vi "Vision Aim 359.vi"(11 "abort":bool) -> (0 "ARM GOOD":bool=TRUE, 1 "WHEELS GOOD":bool, 2 "Vision In Range?":bool=TRUE, 3 "Gyro":dbl=-9.742404543514061 format="%.2f")   [LabVIEW 2015]
uses:
  <vilib>/addons/control/pid/pid.llb/PID Control Input Filter (DBL).vi
  Code/Robot Global Data.vi
  <vilib>/Rock Robotics/WPI/Utilities/WPI_GetSetVariantRefNum.vi
  <vilib>/Rock Robotics/WPI/RobotDrive/WPI_RobotDriveArcadeDrive_Standard(NoSaturation).vi
  <vilib>/addons/control/pid/NI_PID_pid.lvlib
panel:
  out "Enum":T1(ring)
  out "Vision":dbl=-0.01718749999999998 format="%.2f"
  in  "Range 2":dbl=0.03
  in  "Speed 2":dbl=0.4
  in  "Speed 1":dbl=0.55
  in  "Range 1":dbl=0.2
  in  "Vision Tolerance":dbl=0.03
  # "Outputs"
  # "Turning Gains"
  # ".55\n.75\n.45\n.05"
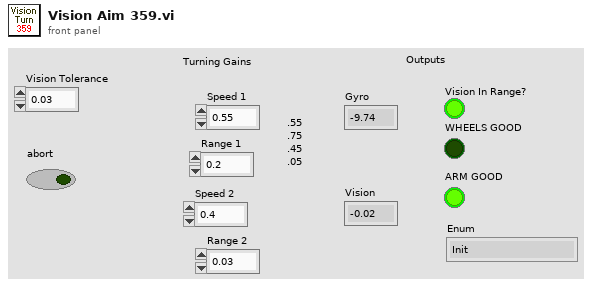
[diagram p1: front panel]
types:
  T1 = enum16{"Init", "Turn Coarse", "Turn Fine ", "Shoot?", "Stop", "Done"}
  T2 = enum16{"Init", "Turn Coarse", "Turn Fine ", "Shoot?", "Stop"}
  T3 = typedef "WPI_RobotDriveDevRef.ctl" = cluster{"DevStatus":errorcluster, "Motors[]":T4[], "Square Inputs":bool, "Max Output":dbl}
  T4 = typedef "WPI_MotorControlDeviceRef.ctl" = cluster{"DeviceStatus":errorcluster, "Type":T5, "PWM":cluster{"PWM Channel":T6, "DeadBand":T7}, "CAN":cluster{"Device Number":u8, "Control Mode":T8, "Semaphore":T9, "Max Vout":dbl, "TalonSRX Control Mode":T10}, "Invert":bool}
  T5 = typedef "WPI_MotorControlType.ctl" = enum16{"PWM", "CAN", "CANTalonSRX"}
  T6 = typedef "FPGA_DIOPWMChannel.ctl" = enum8{"PWM 0", "PWM 1", "PWM 2", "PWM 3", "PWM 4", "PWM 5", "PWM 6", "PWM 7", "PWM 8", "PWM 9", "PWM MXP 0", "PWM MXP 1", "PWM MXP 2", "PWM MXP 3", "PWM MXP 4", "PWM MXP 5", "PWM MXP 6", "PWM MXP 7", "PWM MXP 8", "PWM MXP 9", "Invalid"}
  T7 = typedef "WPI_PWMDeadband.ctl" = cluster{"Name":string, "maxPositivePwm":i32, "minPositivePwm":i32, "centerPwm":i32, "maxNegativePwm":i32, "minNegativePwm":i32, "angularRange":u16}
  T8 = typedef "WPI_CANJaguar_ControlMode.ctl" = enum8{"Percent VBus", "Current", "Speed", "Position", "Voltage"}
  T9 = typedef "Semaphore RefNum" = refnum<k1>
  T10 = typedef "WPI_CANTalonSRX_APIControlMode.ctl" = enum8{"Percent VBus", "Speed", "Position", "Slave", "Unchanged / Invalid", "Voltage Compensation", "Current", "Motion Profile"}
  T11 = typedef "WPI_GyroDevRef.ctl" = cluster{"DevStatus":errorcluster, "Analog Channel":T12, "Offset":dbl, "Gain (VoltsPerDegree/Second)":dbl, "Gyro Type":enum16{"Analog", "XRS450"}, "Handle":i32, "SPI Bus":T13, "Device Found":bool, "Sample Rate":dbl, "Calibrate On Open":bool}
  T12 = typedef "FPGA_AIChannel.ctl" = enum8{"AI 0", "AI 1", "AI 2", "AI 3", "AI MXP 0", "AI MXP 1", "AI MXP 2", "AI MXP 3", "Invalid"}
  T13 = typedef "spi_bus.ctl" = enum16{"SPI On-Board, CS0", "SPI On-Board, CS1", "SPI On-Board, CS2", "SPI On-Board, CS3", "SPI MXP", "Invalid"}
  T14 = enum16{"Init", "Get Angle", "Turn Angle ", "Shoot?", "Stop"}
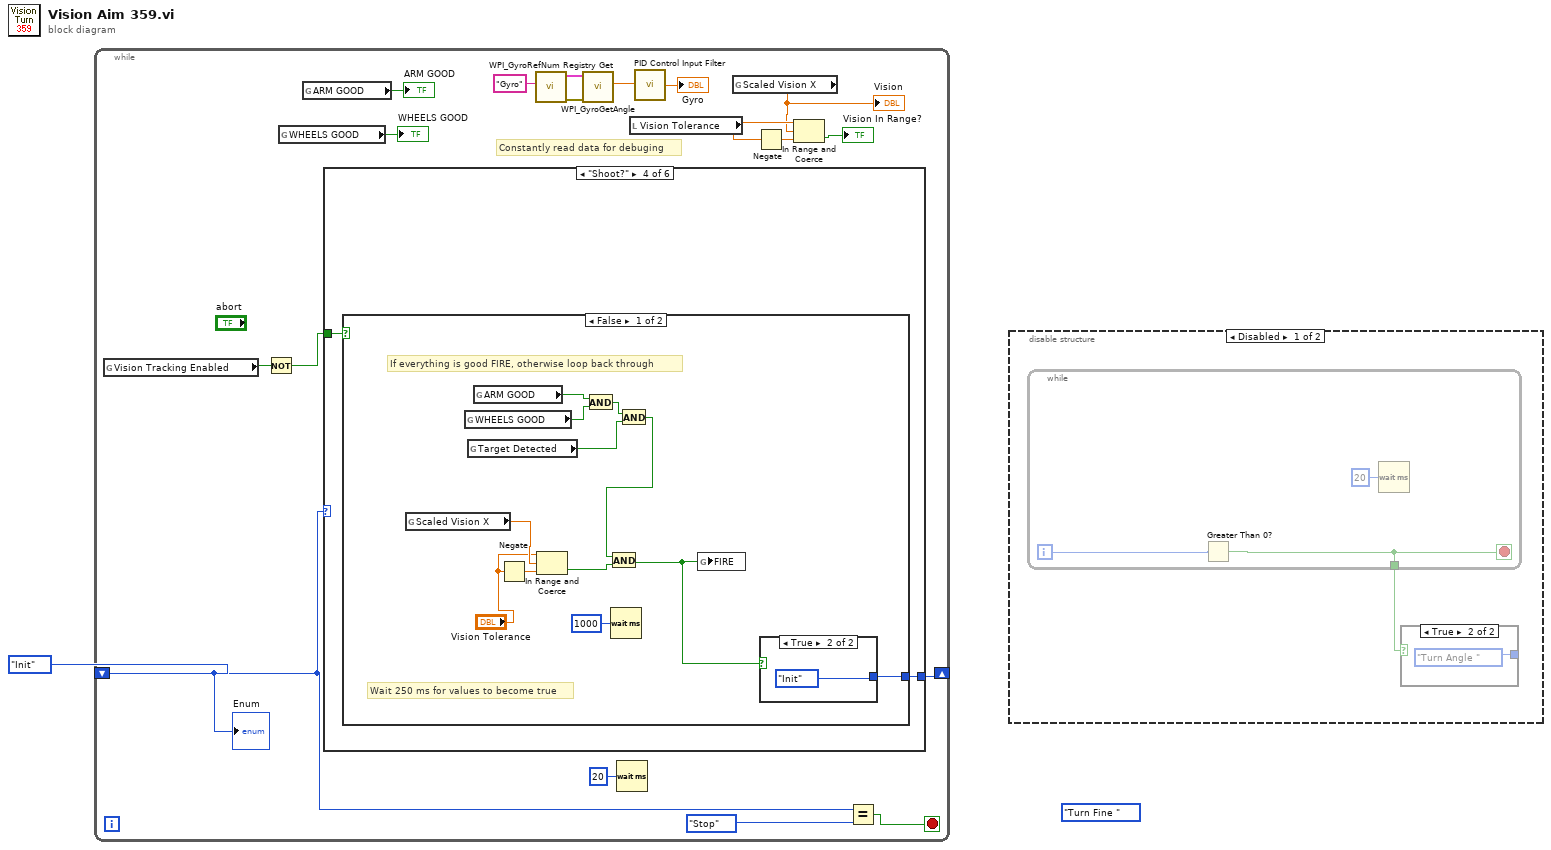
[diagram p0: block diagram]
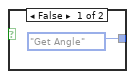
[diagram p2: hidden frame]
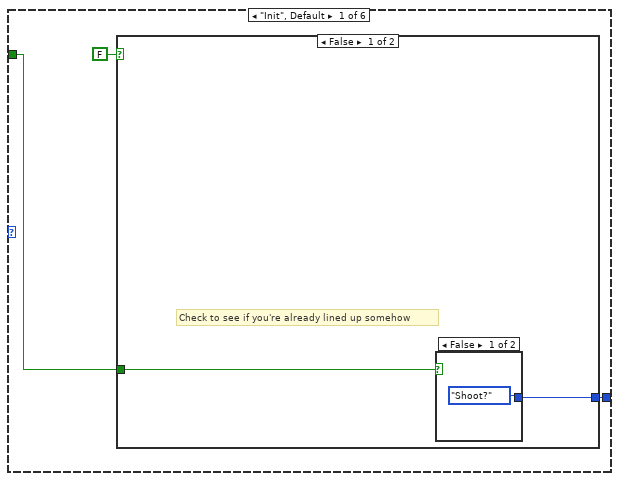
[diagram p4: hidden frame]
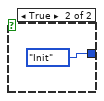
[diagram p5: hidden frame]
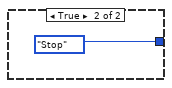
[diagram p6: hidden frame]
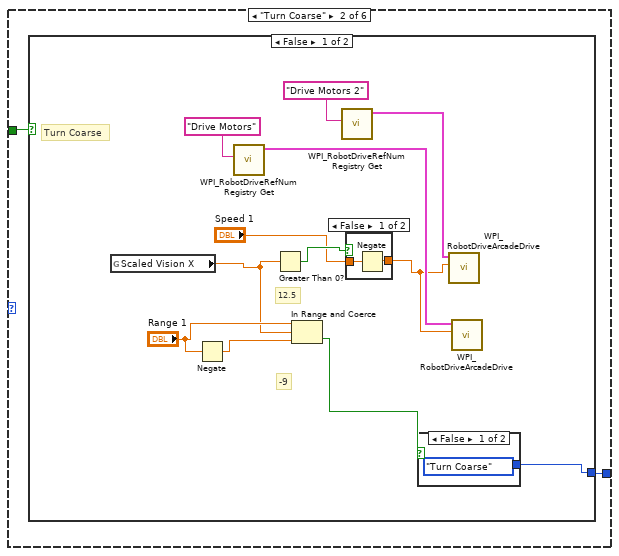
[diagram p7: hidden frame]
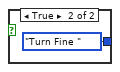
[diagram p8: hidden frame]
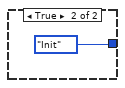
[diagram p10: hidden frame]
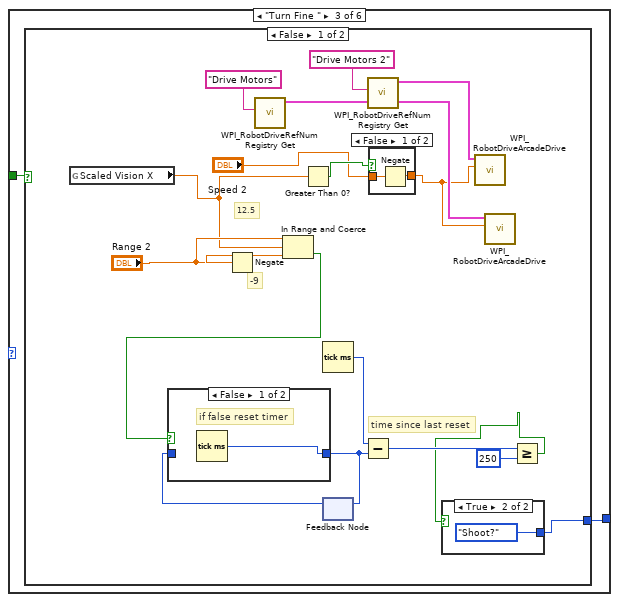
[diagram p11: hidden frame]
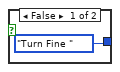
[diagram p12: hidden frame]
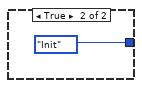
[diagram p15: hidden frame]
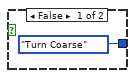
[diagram p16: hidden frame]
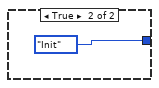
[diagram p17: hidden frame]
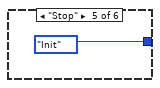
[diagram p18: hidden frame]
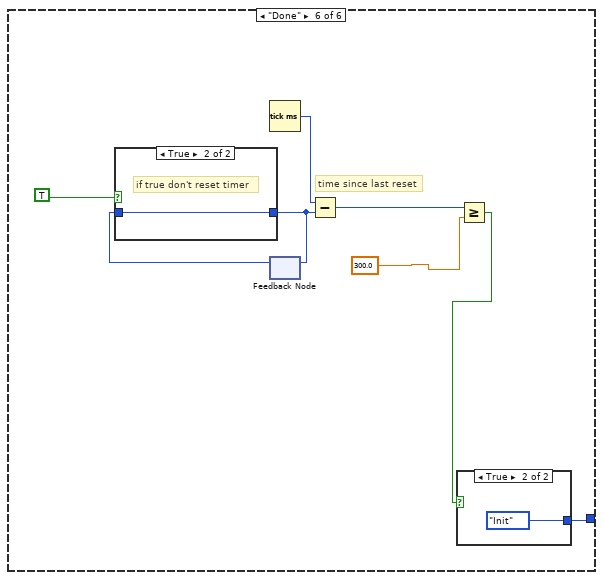
[diagram p19: hidden frame]
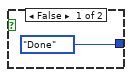
[diagram p20: hidden frame]
diagram:
  (unwired) T2."Turn Fine "
  n1 = while {
    shift-right: [w19] -> _
    shift-left: T1."Init" -> [w17]
    stop <- w18 stop-if-true
    # "Constantly read data for debuging"
    n2 = global read "Robot Global Data.vi" "Vision Tracking Enabled"() -> (w3:bool)
    n3 = Not(x=w3) -> (.not. x?=w2:bool)
    n4 = global read "Robot Global Data.vi" "WHEELS GOOD"() -> (→"WHEELS GOOD":bool)
    n5 = global read "Robot Global Data.vi" "ARM GOOD"() -> (→"ARM GOOD":bool)
    n6 = case shown="\"Shoot?\"" w17 {
      tunnel: w2 -> [w20 w28 w49 w76 _ _]
      tunnel: [w22 w29 w48 w77 T2."Init" w95] -> w19
      frame "Init", Default {
        n7 = case shown="False" FALSE {
          tunnel: [w24 T2."Stop"] -> w22
          tunnel: w20 -> [w23 _]
          frame False {
            # "Check to see if you're already lined up somehow"
            n8 = case shown="False" w23 {
              tunnel: [T1."Shoot?" T1."Init"] -> w24
              frame False {
              }
              frame True {
              }
            }
          }
          frame True {
          }
        }
      }
      frame "Turn Coarse" {
        n9 = case shown="False" w28 {
          tunnel: [w37 T2."Init"] -> w29
          frame False {
            # "-9"
            # "12.5"
            # "Turn Coarse"
            n10 = global read "Robot Global Data.vi" "Scaled Vision X"() -> (w32:dbl)
            n11 = Negate(x="Range 1") -> (-x=w34:dbl)
            n12 = call <vilib>:"WPI_RobotDriveRefNum Registry Get.vi"("refnum name"="Drive Motors") -> ("RobotDriveDevRef"=w40:T3)  [unwired: 1 in, 9 out]
            n13 = Greater Than 0?(x=w32) -> (x > 0?=w36:bool)
            n14 = In Range and Coerce(upper limit="Range 1", x=w32, lower limit=w34) -> (In Range?=w30:bool)  [unwired: 1 out]
            n15 = call <vilib>:"WPI_RobotDriveRefNum Registry Get.vi"("refnum name"="Drive Motors 2") -> ("RobotDriveDevRef"=w38:T3)  [unwired: 1 in, 9 out]
            n16 = case shown="False" w36 {
              tunnel: "Speed 1" -> [w45 w46]
              tunnel: [w44 w46] -> w31
              frame False {
                n17 = Negate(x=w45) -> (-x=w44:dbl)
              }
              frame True {
              }
            }
            n18 = case shown="False" w30 {
              tunnel: [T2."Turn Coarse" T2."Turn Fine "] -> w37
              frame False {
              }
              frame True {
              }
            }
            n19 = call-poly <vilib>:"WPI_RobotDriveArcadeDrive.vi"("X axis value"=w31, "RobotDriveDevRef"=w38) -> ()  [unwired: 7 in, 3 out]
            n20 = call-poly <vilib>:"WPI_RobotDriveArcadeDrive.vi"("X axis value"=w31, "RobotDriveDevRef"=w40) -> ()  [unwired: 7 in, 3 out]
          }
          frame True {
          }
        }
      }
      frame "Turn Fine " {
        n21 = case shown="False" w49 {
          tunnel: [w63 T2."Init"] -> w48
          frame False {
            # "time since last reset"
            # "-9"
            # "12.5"
            n22 = global read "Robot Global Data.vi" "Scaled Vision X"() -> (w58:dbl)
            n23 = Negate(x="Range 2") -> (-x=w61:dbl)
            n24 = call <vilib>:"WPI_RobotDriveRefNum Registry Get.vi"("refnum name"="Drive Motors") -> ("RobotDriveDevRef"=w64:T3)  [unwired: 1 in, 9 out]
            n25 = In Range and Coerce(upper limit="Range 2", x=w58, lower limit=w61) -> (In Range?=w52:bool)  [unwired: 1 out]
            n26 = Greater Than 0?(x=w58) -> (x > 0?=w62:bool)
            n27 = Tick Count (ms)() -> (millisecond timer value=w56:u32)
            n28 = feedback #1() -> (w55:u32)  [unwired: 1 in]
            n29 = case shown="False" w52 {
              tunnel: [w70 w71] -> w54
              tunnel: w55 -> [_ w71]
              frame False {
                # "if false reset timer"
                n30 = Tick Count (ms)() -> (millisecond timer value=w70:u32)
              }
              frame True {
                # "if true don't reset timer"
              }
            }
            n31 = feedback-in #1(w54) -> ()
            n32 = Subtract(x=w56, y=w54) -> (x-y=w53:u32)
            n33 = call <vilib>:"WPI_RobotDriveRefNum Registry Get.vi"("refnum name"="Drive Motors 2") -> ("RobotDriveDevRef"=w65:T3)  [unwired: 1 in, 9 out]
            n34 = case shown="False" w62 {
              tunnel: "Speed 2" -> [w73 w74]
              tunnel: [w72 w74] -> w57
              frame False {
                n35 = Negate(x=w73) -> (-x=w72:dbl)
              }
              frame True {
              }
            }
            n36 = call-poly <vilib>:"WPI_RobotDriveArcadeDrive.vi"("X axis value"=w57, "RobotDriveDevRef"=w65) -> ()  [unwired: 7 in, 3 out]
            n37 = call-poly <vilib>:"WPI_RobotDriveArcadeDrive.vi"("X axis value"=w57, "RobotDriveDevRef"=w64) -> ()  [unwired: 7 in, 3 out]
            n38 = Greater Or Equal?(x=w53, y=u32 250) -> (x >= y?=w50:bool)
            n39 = case shown="True" w50 {
              tunnel: [T2."Turn Fine " T2."Shoot?"] -> w63
              frame False {
              }
              frame True {
              }
            }
          }
          frame True {
          }
        }
      }
      frame "Shoot?" {
        n40 = case shown="False" w76 {
          tunnel: [w89 T2."Init"] -> w77
          frame False {
            # "Wait 250 ms for values to become true"
            # "If everything is good FIRE, otherwise loop back through"
            n41 = global read "Robot Global Data.vi" "Scaled Vision X"() -> (w85:dbl)
            n42 = global read "Robot Global Data.vi" "WHEELS GOOD"() -> (w86:bool)
            n43 = global read "Robot Global Data.vi" "Target Detected"() -> (w79:bool)
            n44 = global read "Robot Global Data.vi" "ARM GOOD"() -> (w87:bool)
            n45 = Negate(x="Vision Tolerance") -> (-x=w83:dbl)
            n46 = In Range and Coerce(upper limit="Vision Tolerance", x=w85, lower limit=w83) -> (In Range?=w88:bool)  [unwired: 1 out]
            n47 = And(x=w87, y=w86) -> (x .and. y?=w80:bool)
            n48 = Wait (ms)(milliseconds to wait=u32 1000) -> ()  [unwired: 1 out]
            n49 = And(x=w80, y=w79) -> (x .and. y?=w78:bool)
            n50 = And(x=w78, y=w88) -> (x .and. y?=w81:bool)
            n51 = global write "Robot Global Data.vi" "FIRE"(w81) -> ()
            n52 = case shown="True" w81 {
              tunnel: [T2."Turn Coarse" T1."Init"] -> w89
              frame False {
              }
              frame True {
              }
            }
          }
          frame True {
          }
        }
      }
      frame "Stop" {
      }
      frame "Done" {
        # "time since last reset"
        n53 = Tick Count (ms)() -> (millisecond timer value=w97:u32)
        n54 = feedback #2() -> (w100:u32)  [unwired: 1 in]
        n55 = case shown="True" TRUE {
          tunnel: [w104 w105] -> w98
          tunnel: w100 -> [_ w105]
          frame False {
            # "if false reset timer"
            n56 = Tick Count (ms)() -> (millisecond timer value=w104:u32)
          }
          frame True {
            # "if true don't reset timer"
          }
        }
        n57 = feedback-in #2(w98) -> ()
        n58 = Subtract(x=w97, y=w98) -> (x-y=w99:u32)
        n59 = Greater Or Equal?(x=w99, y=300.0 ("Delay (ms)")) -> (x >= y?=w94:bool)
        n60 = case shown="True" w94 {
          tunnel: [T1."Done" T1."Init"] -> w95
          frame False {
          }
          frame True {
          }
        }
      }
    }
    n61 = call <vilib>:"WPI_GyroRefNum Registry Get.vi"("refnum name"="Gyro") -> ("error out"=w9:errorcluster, "GyroDevRef"=w8:T11)  [unwired: 9 in]
    n62 = call <vilib>:"WPI_GyroGetAngle.vi"("error in"=w9, "GyroDevRef"=w8) -> ("Angle"=w7:dbl)  [unwired: 5 in, 4 out]
    n63 = Wait (ms)(milliseconds to wait=u32 20) -> ()  [unwired: 1 out]
    n64 = local read "Vision Tolerance"() -> (w15:dbl)
    n65 = call-poly <vilib>:"PID Control Input Filter.vi"("input"=w7) -> ("output"=→"Gyro":dbl)  [unwired: 4 in]
    n66 = global read "Robot Global Data.vi" "Scaled Vision X"() -> (w4:dbl)
    "Vision" <- w4
    n67 = Negate(x=w15) -> (-x=w14:dbl)
    n68 = In Range and Coerce(upper limit=w15, x=w4, lower limit=w14) -> (In Range?=→"Vision In Range?":bool)  [unwired: 1 out]
    n69 = Equal?(x=w17, y=T2."Stop") -> (x = y?=w18:bool)
    "Enum" <- w17
  }
  n70 = disable-structure shown="Disabled" {
    frame Disabled {
      n71 = while {
        tunnel: [w111] -> w106
        i -> [w110]
        stop <- w111 stop-if-true
        n72 = Greater Than 0?(x=w110) -> (x > 0?=w111:bool)
        n73 = Wait (ms)(milliseconds to wait=u32 20) -> ()  [unwired: 1 out]
      }
      n74 = case shown="True" w106 {
        tunnel: [T14."Get Angle" T14."Turn Angle "] -> _
        frame False {
        }
        frame True {
        }
      }
    }
    frame Enabled {
    }
  }
